vi "多个线圈写入.vi"(8 "Error in":errorcluster caption="Error in (no error)", 9 "values":bool[](array[boolean]), 10 "starting address":u16, 11 "Slave ID":u8=10) -> (0 "error out":errorcluster)   [LabVIEW 2016, in "质控单元.lvlib"]
uses:
  <vilib>/Plasmionique/MB Master/MB_Master_TCP/MB_Master_TCP.lvclass
  D:/Program Files (x86)/National Instruments/LabVIEW 2016/vi.lib/Plasmionique/MB Master/MB_Master/MB_Master.lvclass
  <vilib>/Plasmionique/MB Master/MB_Master/MB_Master.lvclass
  <vilib>/Plasmionique/MB Master/MB Master.lvlib
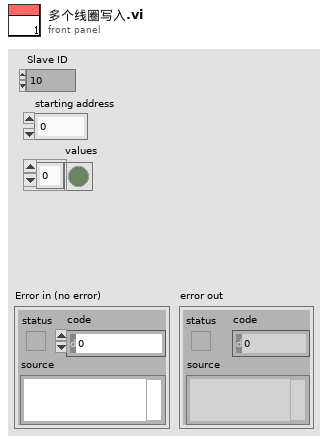
[diagram p1: front panel]
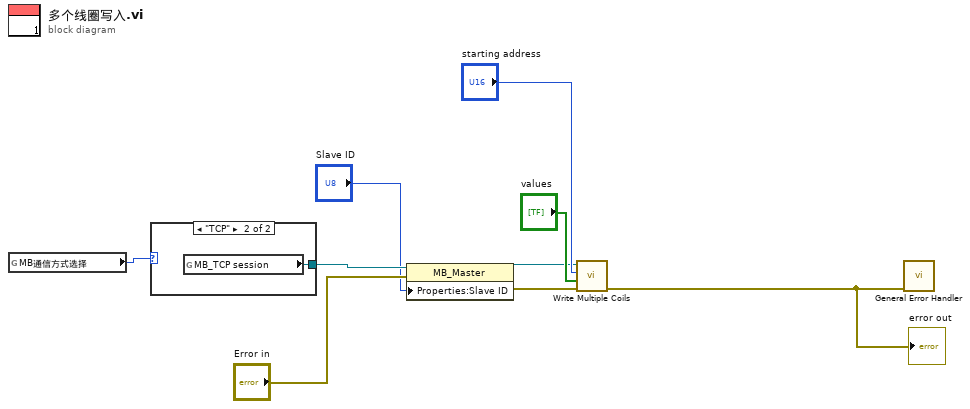
[diagram p0: block diagram]
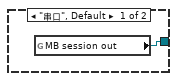
[diagram p2: hidden frame]
diagram:
  n1 = global read "断电保存全局.vi" "MB通信方式选择"() -> (w7:enum16{"串口", "TCP"})
  n2 = case shown="\"TCP\"" w7 {
    tunnel: [w10 w11] -> w6
    frame "串口", Default {
      n3 = global read "断电保存全局.vi" "MB session out"() -> (w10:refnum<class "MB_Master.lvclass">)
    }
    frame "TCP" {
      n4 = global read "断电保存全局.vi" "MB_TCP session"() -> (w11:refnum<class "MB_Master_TCP.lvclass">)
    }
  }
  n5 = property class="MB_Master"(reference=w6, error in="Error in", "Properties:Slave ID"="Slave ID") -> (reference out=w5:refnum<class "MB_Master.lvclass">, error out=w4:errorcluster)
  n6 = call <vilib>:"Write Multiple Coils.vi"("error in (no error)"=w4, "values"="values", "starting address"="starting address", "MB session in"=w5) -> ("error out"=w2:errorcluster)  [unwired: 6 in, 1 out]
  "error out" <- w2
  n7 = call <vilib>:"General Error Handler.vi"("error in (no error)"=w2) -> ()  [unwired: 10 in, 5 out]
